vi "Main.vi"(8 "error in":errorcluster, 10 "Sequence Context":refnum<k7>, 11 "PreUUT In":refnum<class "PreUUT.lvclass">) -> (0 "error out":errorcluster, 3 "PreUUT Out":refnum<class "PreUUT.lvclass">)   [LabVIEW 2019, in "Sequence Main.lvlib" / "PreUUT.lvclass"]
uses:
  PreUUT.lvclass
  C:/Workspace/gip-fct/Sequence/CodeModules/PreTestPost Launcher/Abstract UUT/Abstract UUT.lvclass
  PreUUT.lvclass/PreUUT.ctl
  Abstract UUT/Abstract UUT.lvclass
panel:
  in  "Barcode":string
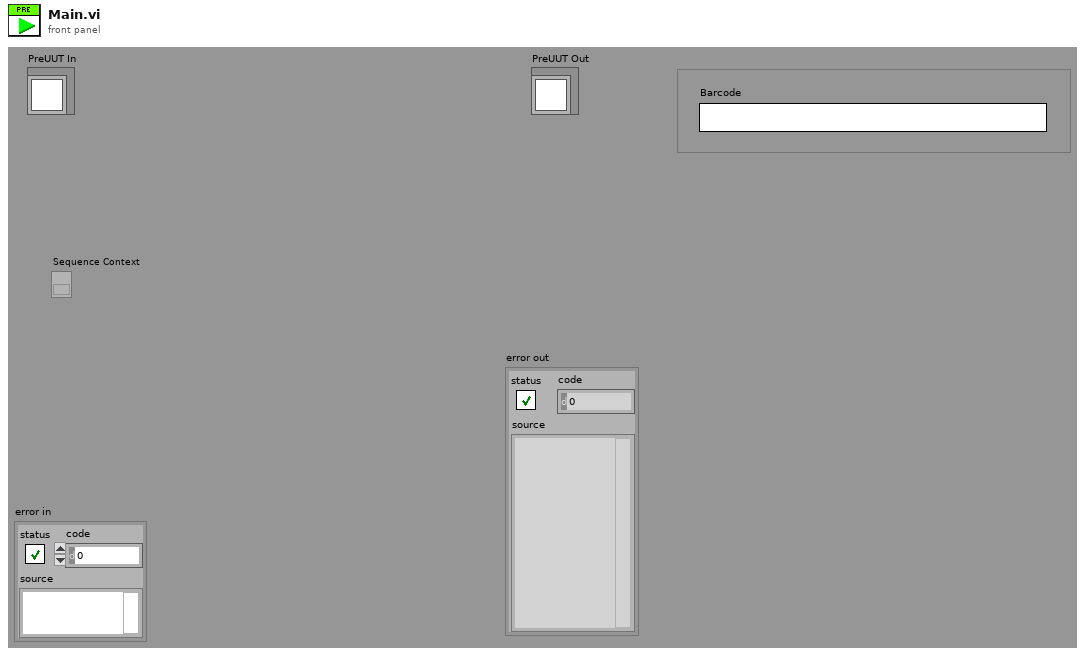
[diagram p1: front panel]
types:
  T1 = typedef "TestStand - Status Monitor.ctl" = cluster{"Sequence Context":refnum<k7>, "Execution":refnum<k7>, "Termination Monitor":refnum<k7>}
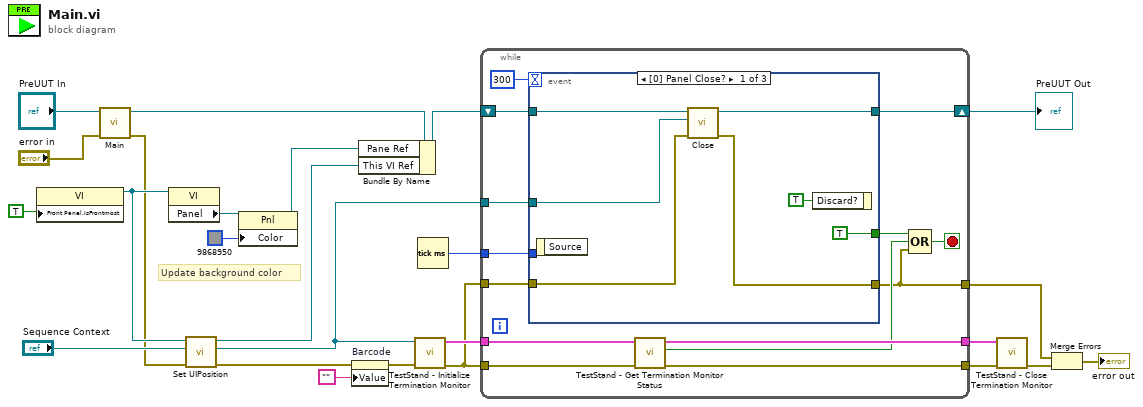
[diagram p0: block diagram]
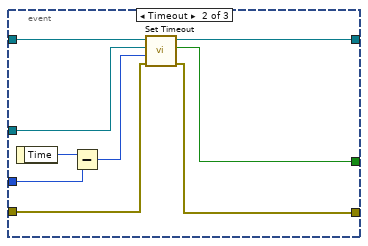
[diagram p2: hidden frame]
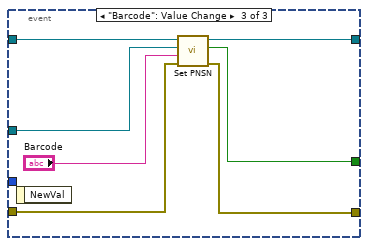
[diagram p3: hidden frame]
diagram:
  # "Update background color"
  n1 = property class="VI"("Front Panel.IsFrontmost"=TRUE ("Front Panel Window:Is Frontmost")) -> (reference out=w11:refnum<vi>)  [unwired: 2 in, 1 out]
  n2 = call-parent "Main.vi"("error in"="error in", "OPC UA In"="PreUUT In") -> ("error out"=w9:errorcluster, "OPC UA Out"=w15:refnum<class "PreUUT.lvclass">)  [unwired: 8 in]
  n3 = property class="VI"(reference=w11) -> ("Panel"=w23:refnum<vi>)  [unwired: 1 in, 2 out]
  n4 = call "Set UIPosition.vi"("error in"=w9, "Sequence Context In"="Sequence Context", "VI Ref"=w11) -> ("error out"=w3:errorcluster, "Sequence Context out"=w4:refnum<k7>, "VI Ref out"=w10:refnum<vi>)  [unwired: 6 in]
  n5 = property class="Pnl"(reference=w23, "Color"=u32 9868950 ("Color Box")) -> (reference out=w13:refnum<vi>)  [unwired: 1 in, 1 out]
  n6 = property on="Barcode" class="Str"(error in=w3, "Value"="") -> (error out=w2:errorcluster)  [unwired: 1 in, 1 out]
  n7 = Bundle By Name(cluster=w15, "Pane Ref"=w13, "This VI Ref"=w10) -> (w14:refnum<class "PreUUT.lvclass">)
  n8 = call <vilib>:"TestStand - Initialize Termination Monitor.vi"("error in (no error)"=w2, "Sequence Context In"=w4) -> ("error out"=w8:errorcluster, "Status Monitor Out"=w22:T1)  [unwired: 8 in]
  n9 = Tick Count (ms)() -> (millisecond timer value=w5:u32)
  n10 = while {
    tunnel: w8 -> [w37]
    tunnel: w22 -> [w36]
    tunnel: [w30] -> w21
    tunnel: [w34] -> w20
    tunnel: w8 -> [w29]
    tunnel: [w28] -> w6
    tunnel: w5 -> [w27]
    shift-right: [w33] -> w19
    shift-left: w14 -> [w39]
    tunnel: w4 -> [w26]
    stop <- w35 stop-if-true
    n11 = event shown="[0] Panel Close?" {
      selector: _ -> [_ _ _]
      dyn-events: _ -> [_ _ _]
      timeout: 300 -> [_ _ _]
      tunnel: w39 -> [w44 w53 w62]
      tunnel: [w43 w47 w61] -> w33
      tunnel: [TRUE ("Stop") w49 w60] -> w31
      tunnel: w29 -> [w42 w51 w59]
      tunnel: [w41 w50 w58] -> w28
      tunnel: w27 -> [_ w54 _]
      tunnel: w26 -> [w40 w48 w57]
      event Panel Close? {
        n12 = event-data() -> ()  [unwired: 1 in, 1 out]
        n13 = call-dynamic "Close.vi"("error in (no error)"=w42, "Sequence Context"=w40, "PreUUT in"=w44) -> ("error out"=w41:errorcluster, "PreUUT out"=w43:refnum<class "PreUUT.lvclass">)  [unwired: 7 in]
        n14 = event-data("Discard?"=TRUE) -> ()  [unwired: 1 in, 1 out]
      }
      event Timeout {
        n15 = event-data() -> ("Time"=w55:u32)  [unwired: 1 in]
        n16 = Subtract(x=w55, y=w54) -> (x-y=w52:u32)
        n17 = call "Set Timeout.vi"("error in (no error)"=w51, "Elapsed Time"=w52, "Sequence Context"=w48, "Abstract UUT in"=w53) -> ("error out"=w50:errorcluster, "Timeout"=w49:bool, "Abstract UUT out"=w47:refnum<class "PreUUT.lvclass">)  [unwired: 5 in]
      }
      event "Barcode": Value Change {
        n18 = event-data() -> ()  [unwired: 1 in, 1 out]
        n19 = call "Set PNSN.vi"("error in"=w59, "Barcode"="Barcode", "Sequence Context"=w57, "PreUUT in"=w62) -> ("error out"=w58:errorcluster, "Found?"=w60:bool, "PreUUT out"=w61:refnum<class "PreUUT.lvclass">)  [unwired: 5 in]
      }
    }
    n20 = call <vilib>:"TestStand - Get Termination Monitor Status.vi"("error in (no error)"=w37, "Status Monitor In"=w36) -> ("error out"=w30:errorcluster, "Terminating or Aborting"=w32:bool, "Status Monitor Out"=w34:T1)  [unwired: 7 in]
    n21 = Compound Arithmetic op=OR(w31, w32, w28) -> (w35:bool)
  }
  "PreUUT Out" <- w19
  n22 = call <vilib>:"TestStand - Close Termination Monitor.vi"("error in (no error)"=w21, "Status Monitor In"=w20) -> ("error out"=w16:errorcluster)  [unwired: 9 in]
  n23 = Merge Errors(w6, w16) -> (→"error out":errorcluster)
